vi "Names to colors for twin paper.vi"(11 "Plot Names 2":string[][](array[string])) -> (2 "Line Styles":u8[](array[numeric]), 3 "Plot Colors":u32[](array[colorbox])=[16711680, 9896136, 16772608, 26111, 56357, 0])   [LabVIEW 2010]
uses:
  <vilib>/regexp/Match Regular Expression.xnode
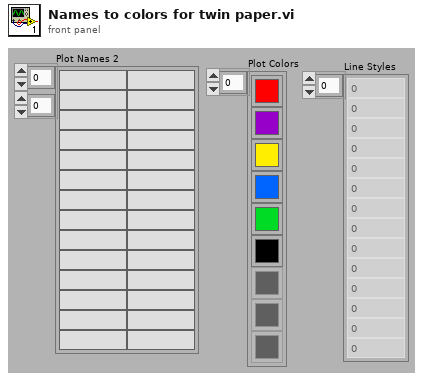
[diagram p1: front panel]
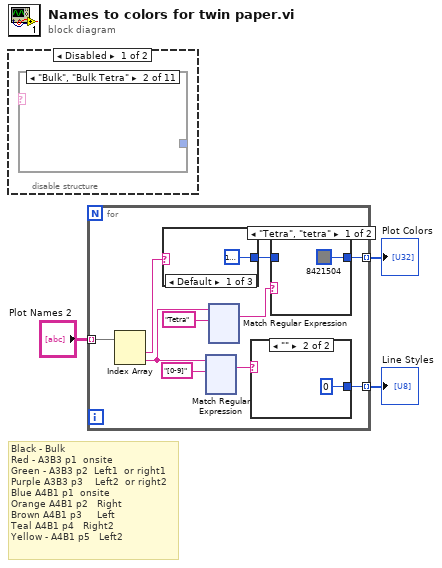
[diagram p0: block diagram]
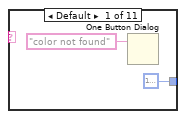
[diagram p2: hidden frame]
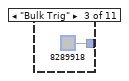
[diagram p3: hidden frame]
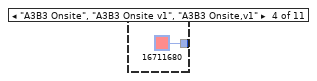
[diagram p4: hidden frame]
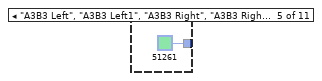
[diagram p5: hidden frame]
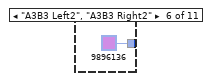
[diagram p6: hidden frame]
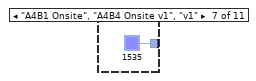
[diagram p7: hidden frame]
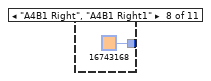
[diagram p8: hidden frame]
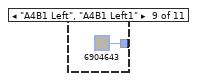
[diagram p9: hidden frame]
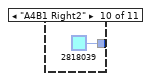
[diagram p10: hidden frame]
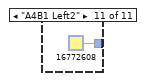
[diagram p11: hidden frame]
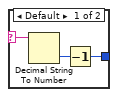
[diagram p14: hidden frame]
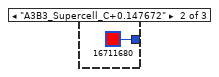
[diagram p15: hidden frame]
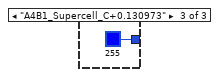
[diagram p16: hidden frame]
diagram:
  # "Black - Bulk\nRed - A3B3 p1  onsite\nGreen - A3B3 p2  Left1  or right1\nPurple A3B3 p3    Left2  or right2\nBlue A4B1 p1  onsite\nOrange A4B1 p2   Right\nBrown A4B1 p3     Left\nTeal A4B1 p4   Right2\nYellow - A4B1 p5   Left2"
  n1 = disable-structure shown="Disabled" {
    frame Disabled {
      n2 = case shown="\"Bulk\", \"Bulk Tetra\"" {
        selector: _ -> [_ _ _ _ _ _ _ _ _ _ _]
        tunnel: [u32 16777216 ("Color Box") _ u32 8289918 ("Color Box") u32 16711680 ("Color Box") u32 51261 ("Color Box") u32 9896136 ("Color Box") u32 1535 ("Color Box") u32 16743168 ("Color Box") u32 6904643 ("Color Box") u32 2818039 ("Color Box") u32 16772608 ("Color Box")] -> _
        frame Default {
          n3 = One Button Dialog(message="color not found") -> ()  [unwired: 1 in, 1 out]
        }
        frame "Bulk", "Bulk Tetra" {
        }
        frame "Bulk Trig" {
        }
        frame "A3B3 Onsite", "A3B3 Onsite v1", "A3B3 Onsite,v1" {
        }
        frame "A3B3 Left", "A3B3 Left1", "A3B3 Right", "A3B3 Right1" {
        }
        frame "A3B3 Left2", "A3B3 Right2" {
        }
        frame "A4B1 Onsite", "A4B4 Onsite v1", "v1" {
        }
        frame "A4B1 Right", "A4B1 Right1" {
        }
        frame "A4B1 Left", "A4B1 Left1" {
        }
        frame "A4B1 Right2" {
        }
        frame "A4B1 Left2" {
        }
      }
    }
    frame Enabled {
    }
  }
  n4 = for {
    tunnel: "Plot Names 2" -> [w24] mode=indexing
    tunnel: [w15] -> w3 mode=indexing
    tunnel: [w20] -> w1 mode=indexing
    n5 = Index Array(array=w24) -> (element #1=w23:string, element #2=w19:string)  [unwired: 2 in]
    n6 = case shown="Default" w23 {
      tunnel: [u32 16777222 ("Color Box") u32 16711680 ("Color Box") u32 255 ("Color Box")] -> w16
      frame Default {
      }
      frame "A3B3_Supercell_C+0.147672" {
      }
      frame "A4B1_Supercell_C+0.130973" {
      }
    }
    n7 = xnode "Match Regular Expression"("input string"=w19, "regular expression"="[0-9]") -> ("whole match"=w21:string)  [unwired: 4 in, 4 out]
    n8 = xnode "Match Regular Expression"("input string"=w19, "regular expression"="Tetra") -> ("whole match"=w17:string)  [unwired: 4 in, 4 out]
    n9 = case shown="\"\"" w21 {
      selector: w21 -> [w251 _]
      tunnel: [w249 0] -> w20
      frame Default {
        n10 = Decimal String To Number(string=w251) -> (number=w250:i32)  [unwired: 2 in, 1 out]
        n11 = Decrement(x=w250) -> (x-1=w249:i32)
      }
      frame "" {
      }
    }
    n12 = case shown="\"Tetra\", \"tetra\"" w17 {
      tunnel: [u32 8421504 ("Color Box") w26] -> w15
      tunnel: w16 -> [_ w26]
      frame "Tetra", "tetra" {
      }
      frame "", Default {
      }
    }
  }
  "Plot Colors" <- w3
  "Line Styles" <- w1
